vi "Test Longer than Target.vi"(11 "Test Case In":refnum<class "Common Chars Finder Test.lvclass">) -> (0 "error out":errorcluster, 3 "Test Case Out":refnum<class "Common Chars Finder Test.lvclass">)   [LabVIEW 2020, in "Common Chars Finder Test.lvclass"]
uses:
  Common Chars Finder Test.lvclass
  usr/local/natinst/LabVIEW-2026-64/vi.lib/Astemes/LUnit/Test Case.lvclass
  <vilib>/Astemes/LUnit/Test Case.lvclass/Test Case.ctl
  4993e8ee-a06a-463a-9684-69129f64d5ce.vi
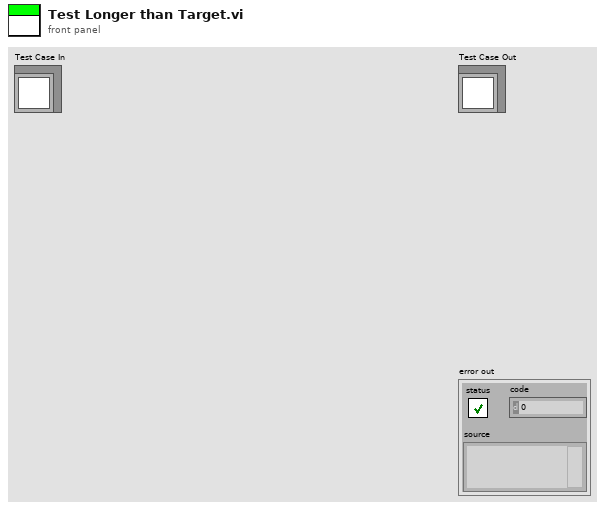
[diagram p1: front panel]
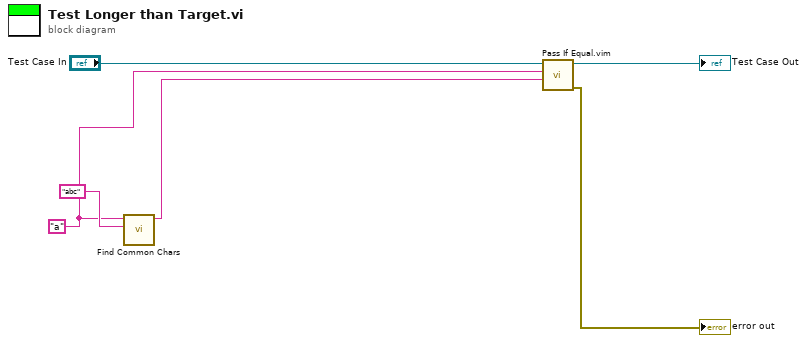
[diagram p0: block diagram]
diagram:
  w1 = "a" ("Reference")
  n1 = call "Find Common Chars.vi"("Reference"="abc" ("Target"), "Target"=w1) -> ("Common"=w2:string)  [unwired: 9 in]
  n2 = call "Pass If Equal.vim"("Actual"=w2, "Expected"=w1, "LUnit Test Case In"="Test Case In") -> ("error out"=→"error out":errorcluster, "LUnit Test Case Out"=→"Test Case Out":refnum<class "Common Chars Finder Test.lvclass">)  [unwired: 7 in]
